vi "Wheel Angle From Encoder.vi"(11 "Numeric in":i32) -> (3 "Numeric out":dbl)   [LabVIEW 2014]
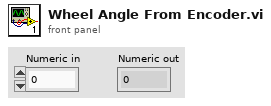
[diagram p1: front panel]
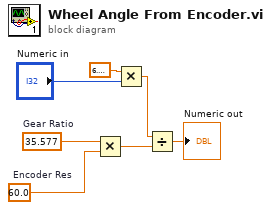
[diagram p0: block diagram]
diagram:
  w4 = 60.0  # Encoder Res
  w3 = 35.577  # Gear Ratio
  n1 = Multiply(x=w3, y=w4) -> (x*y=w6:dbl)
  n2 = Multiply(x=6.283185307179586, y="Numeric in") -> (x*y=w5:dbl)
  n3 = Divide(x=w5, y=w6) -> (x/y=→"Numeric out":dbl)
